vi "Network Write.vi"(7 "Values":dbl[](array[numeric]), 8 "error in (no error)":errorcluster, 10 "RDB References in":T4 {"RDB Send Reference"."RDB Data"."payload" format="%x"; "RDB Send Reference"."RDB Data"."timestamp" format="%<%.7X\n%x>T"; "RDB Send Reference"."RDB Data"."type" items=["FlexRay Data"=32, "FlexRay Null"=33, "FlexRay Symbol"=34, "Log Trigger"=225, "Start Trigger"=226]; "RDB Send Reference"."RDB Data"."cycle count" max=63 step=1; "RDB Receive Reference"."RDB Data"."payload" format="%x"; "RDB Receive Reference"."RDB Data"."timestamp" format="%<%.7X\n%x>T"; "RDB Receive Reference"."RDB Data"."type" items=["FlexRay Data"=32, "FlexRay Null"=33, "FlexRay Symbol"=34, "Log Trigger"=225, "Start Trigger"=226]; "RDB Receive Reference"."RDB Data"."cycle count" max=63 step=1}, 11 "Settings":T1={"UDP Receiver"=refnum, "UDP Sender"=refnum, "Valid Packet"=FALSE, "TCP"=refnum, "Network Settings"={"IP adress"="127.0.0.1", "RDB"={"Protocol"=enum."UDP", "Tx Port"=48270, "Rx Port"=10, "Buffer Size"=204800, "Timeout"=10}, "SCP"={"Protocol"=enum."TCP", "Tx Port"=48191, "Rx Port"=48191, "Buffer Size"=204800, "Timeout"=10}}, "vclient"=path ""}) -> (0 "error out":errorcluster, 2 "RDB Reference out":T4 {"RDB Send Reference"."RDB Data"."payload" format="%x"; "RDB Send Reference"."RDB Data"."timestamp" format="%<%.7X\n%x>T"; "RDB Send Reference"."RDB Data"."type" items=["FlexRay Data"=32, "FlexRay Null"=33, "FlexRay Symbol"=34, "Log Trigger"=225, "Start Trigger"=226]; "RDB Send Reference"."RDB Data"."cycle count" max=63 step=1; "RDB Receive Reference"."RDB Data"."payload" format="%x"; "RDB Receive Reference"."RDB Data"."timestamp" format="%<%.7X\n%x>T"; "RDB Receive Reference"."RDB Data"."type" items=["FlexRay Data"=32, "FlexRay Null"=33, "FlexRay Symbol"=34, "Log Trigger"=225, "Start Trigger"=226]; "RDB Receive Reference"."RDB Data"."cycle count" max=63 step=1}, 3 "Settings":T1={"UDP Receiver"=refnum, "UDP Sender"=refnum, "Valid Packet"=FALSE, "TCP"=refnum, "Network Settings"={"IP adress"="127.0.0.1", "RDB"={"Protocol"=enum."UDP", "Tx Port"=48270, "Rx Port"=10, "Buffer Size"=204800, "Timeout"=10}, "SCP"={"Protocol"=enum."TCP", "Tx Port"=48191, "Rx Port"=48191, "Buffer Size"=204800, "Timeout"=10}}, "vclient"=path ""})   [LabVIEW 2020, in "Vires VTD Engine.lvlib"]
uses:
  Vires VTD Engine.lvlib
  RDB/RDB References.ctl
  RDB/RDB Reference.ctl
  <vilib>/xnet/xnet.llb/XNET Frame FlexRay.ctl
  <vilib>/xnet/xnet.llb/XNET Frame Type FlexRay.ctl
  Type/Settings.ctl
  Shared/Network Settings.ctl
  Shared/Protocol.ctl
  RDB/RDB.lvlib
  Shared/Vires VTD Shared.lvlib
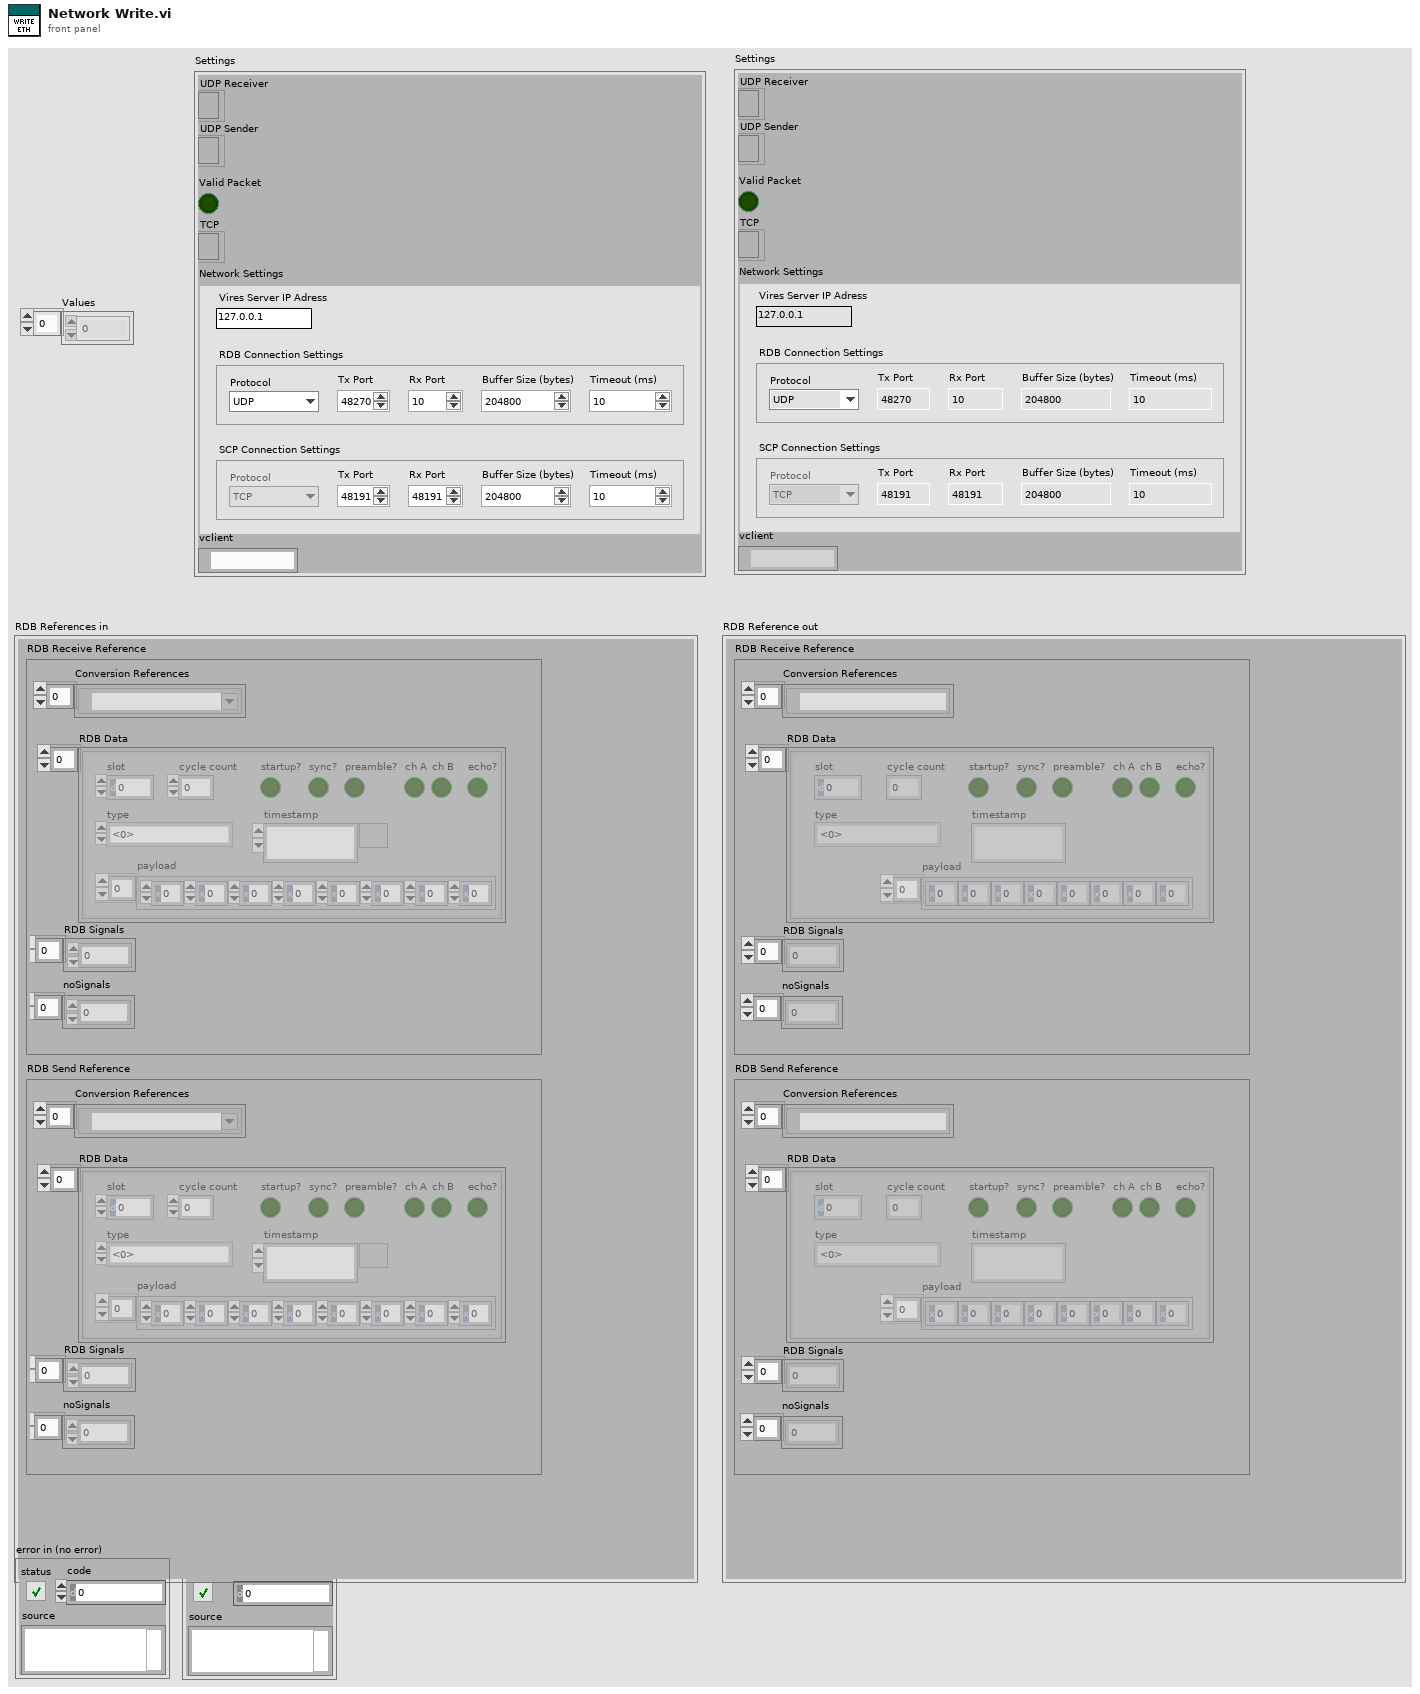
[diagram p1: front panel]
types:
  T1 = typedef "Vires VTD Engine.lvlib/Settings.ctl" = cluster{"UDP Receiver":refnum<k16>, "UDP Sender":refnum<k16>, "Valid Packet":bool, "TCP":refnum<k5>, "Network Settings":T2, "vclient":path}
  T2 = typedef "Vires VTD Shared.lvlib/Network Settings.ctl" = cluster{"IP adress":string, "RDB":cluster{"Protocol":T3, "Tx Port":u16, "Rx Port":u16, "Buffer Size":i32, "Timeout":u16}, "SCP":cluster{"Protocol":T3, "Tx Port":u16, "Rx Port":u16, "Buffer Size":i32, "Timeout":u16}}
  T3 = typedef "Vires VTD Shared.lvlib/Protocol.ctl" = enum16{"UDP", "TCP"}
  T4 = typedef "RDB.lvlib/RDB References.ctl" = cluster{"RDB Receive Reference":T5, "RDB Send Reference":T5}
  T5 = typedef "RDB.lvlib/RDB Reference.ctl" = cluster{"Conversion References":refnum<k21>[], "RDB Data":T6[], "RDB Signals":dbl[], "noSignals":i32[]}
  T6 = typedef "XNET Frame FlexRay.ctl" = cluster{"timestamp":timestamp, "payload":u8[], "slot":u16, "type":T7, "cycle count":u8, "startup?":bool, "sync?":bool, "preamble?":bool, "ch A":bool, "ch B":bool, "echo?":bool}
  T7 = typedef "XNET Frame Type FlexRay.ctl" = u8
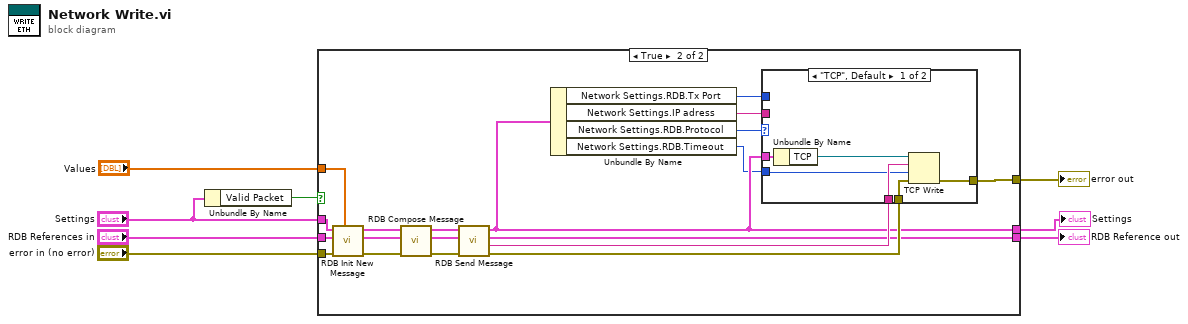
[diagram p0: block diagram]
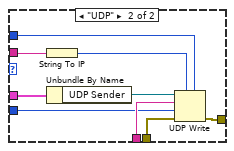
[diagram p3: hidden frame]
diagram:
  n1 = Unbundle By Name("Settings") -> ("Valid Packet"=w4:bool)
  n2 = case shown="True" w4 {
    tunnel: [w11 w29] -> w8
    tunnel: [w10 w15] -> w7
    tunnel: "error in (no error)" -> [w11 w24]
    tunnel: "Values" -> [_ w23]
    tunnel: "RDB References in" -> [w10 w16]
    tunnel: "Settings" -> [w9 w14]
    tunnel: [w9 w13] -> w1
    frame False {
    }
    frame True {
      n3 = call "RDB Init New Message.vi"("RDB Receive Reference.RDB Signals"=w23, "error in (no error)"=w24, "RDB Reference in"=w16, "Settings"=w14) -> ("error out"=w25:errorcluster, "RDB Reference out"=w17:T4, "Settings"=w30:T1)  [unwired: 5 in]
      n4 = call "RDB Compose Message.vi"("error in (no error)"=w25, "RDB Reference in"=w17, "Settings"=w30) -> ("error out"=w26:errorcluster, "RDB Reference out"=w18:T4, "Settings"=w27:T1)  [unwired: 6 in]
      n5 = call "RDB Send Message.vi"("error in (no error)"=w26, "RDB Reference in"=w18, "Settings"=w27) -> ("error out"=w28:errorcluster, "RDB Message"=w19:string, "RDB Reference out"=w15:T4, "Settings"=w13:T1)  [unwired: 5 in]
      n6 = Unbundle By Name(w13) -> ("Network Settings.RDB.Tx Port"=w20:u16, "Network Settings.IP adress"=w21:string, "Network Settings.RDB.Protocol"=w22:T3, "Network Settings.RDB.Timeout"=w12:u16)
      n7 = case shown="\"TCP\", Default" w22 {
        tunnel: w19 -> [w32 w44]
        tunnel: [w33 w43] -> w29
        tunnel: w28 -> [w34 w42]
        tunnel: w13 -> [w36 w40]
        tunnel: w21 -> [_ w39]
        tunnel: w20 -> [_ w38]
        tunnel: w12 -> [w31 w37]
        frame "TCP", Default {
          n8 = Unbundle By Name(w36) -> ("TCP"=w35:refnum<k5>)
          n9 = TCP Write(connection ID=w35, data in=w32, error in (no error)=w34, 9:w31) -> (error out=w33:errorcluster)  [unwired: 2 out]
        }
        frame "UDP" {
          n10 = String To IP(1:w39) -> (0:w45:u32)
          n11 = Unbundle By Name(w40) -> ("UDP Sender"=w41:refnum<k16>)
          n12 = UDP Write(address=w45, port or service name=w38, connection ID=w41, data in=w44, 8:w42, 9:w37) -> (error out=w43:errorcluster)  [unwired: 1 out]
        }
      }
    }
  }
  "error out" <- w8
  "RDB Reference out" <- w7
  "Settings" <- w1
